vi "Allan Variance Chart.vi"   [LabVIEW 2021, in "IMU Processing.lvlib" / "ErrorModellingLibrary.lvlib"]
uses:
  ErrorModellingLibrary.lvlib
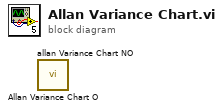
[diagram p0: block diagram]
diagram:
  n1 = call "Allan Variance Chart O.vi"() -> ()  [unwired: 9 in, 3 out]
  n2 = call "allan Variance Chart NO.vi"() -> ()  [unwired: 9 in, 3 out]
